vi "Print Main Screen.vi"(4 "Sample Rate in":T2=enum."500 Hz", 6 "Trigger Type in":T3(ring)=enum."Timed", 8 "Axis Names":string[](array[string]), 10 "Header Information in":T1, 11 "Graph Ref in":refnum<vi>) -> ()   [LabVIEW 2019]
uses:
  Type Defs and Controls/Header Information.ctl
  Type Defs and Controls/Sample Rates.ctl
panel:
  out "Time":string
  out "Date":string
  out "Legend":string[](array[string])
  out "Header Information":T1
  out "Sample Rate":T2=enum."500 Hz"
  out "Trigger Type":T3(ring)=enum."Timed"
  out "Graph":sgl[][](graph)
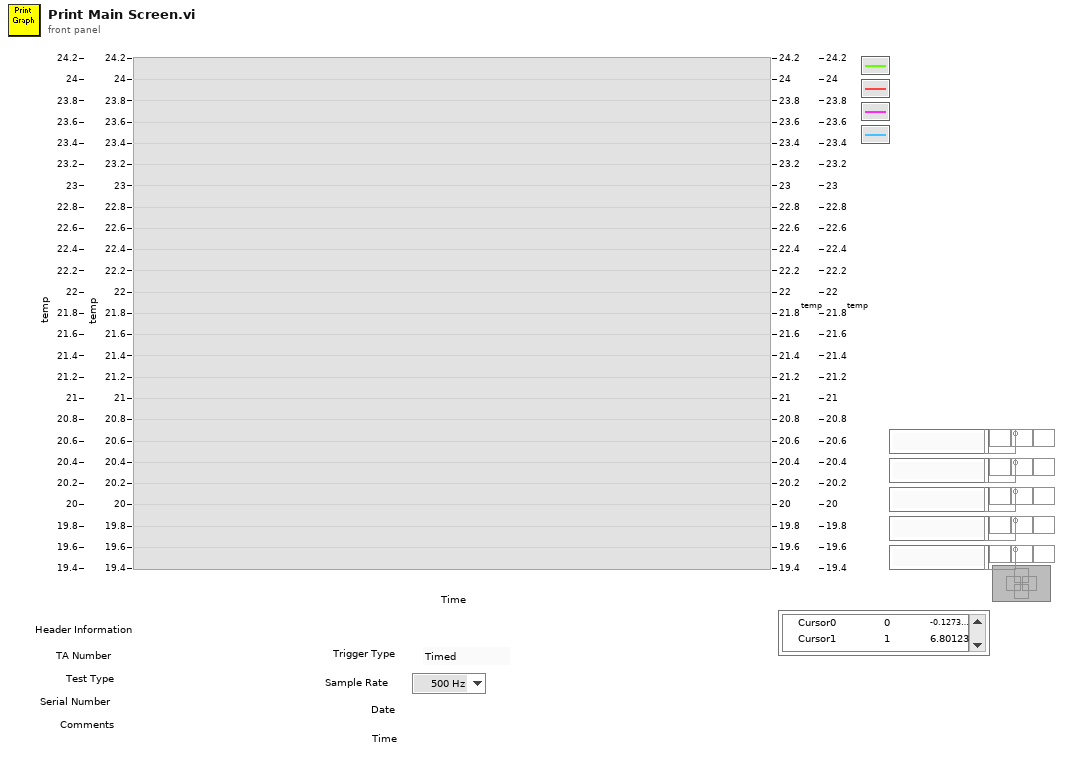
[diagram p1: front panel]
types:
  T1 = typedef "Header Information.ctl" = cluster{"TA Number":string, "Test Type":string, "Serial Number":string, "Comments":string}
  T2 = typedef "Sample Rates.ctl" = enum16{"2000 Hz", "1500 Hz", "1000 Hz", "500 Hz", "200 Hz", "100 Hz", "50 Hz", "25 Hz", "10 Hz", "1 Hz"}
  T3 = enum16{"Manual", "Timed", "Analog Rising", "Analog Falling"}
  T4 = typedef "LVFormatAndPrecisionTypeDef.ctl" = cluster{"Format":u8, "Precision":u8}
  T5 = typedef "LVRangeTypeDef.ctl" = cluster{"Minimum":dbl, "Maximum":dbl, "Increment":dbl, "Minor Increment":dbl, "Start":dbl}
  T6 = typedef "LVPointDoubleTypeDef.ctl" = cluster{"Cursor X":dbl, "Cursor Y":dbl}
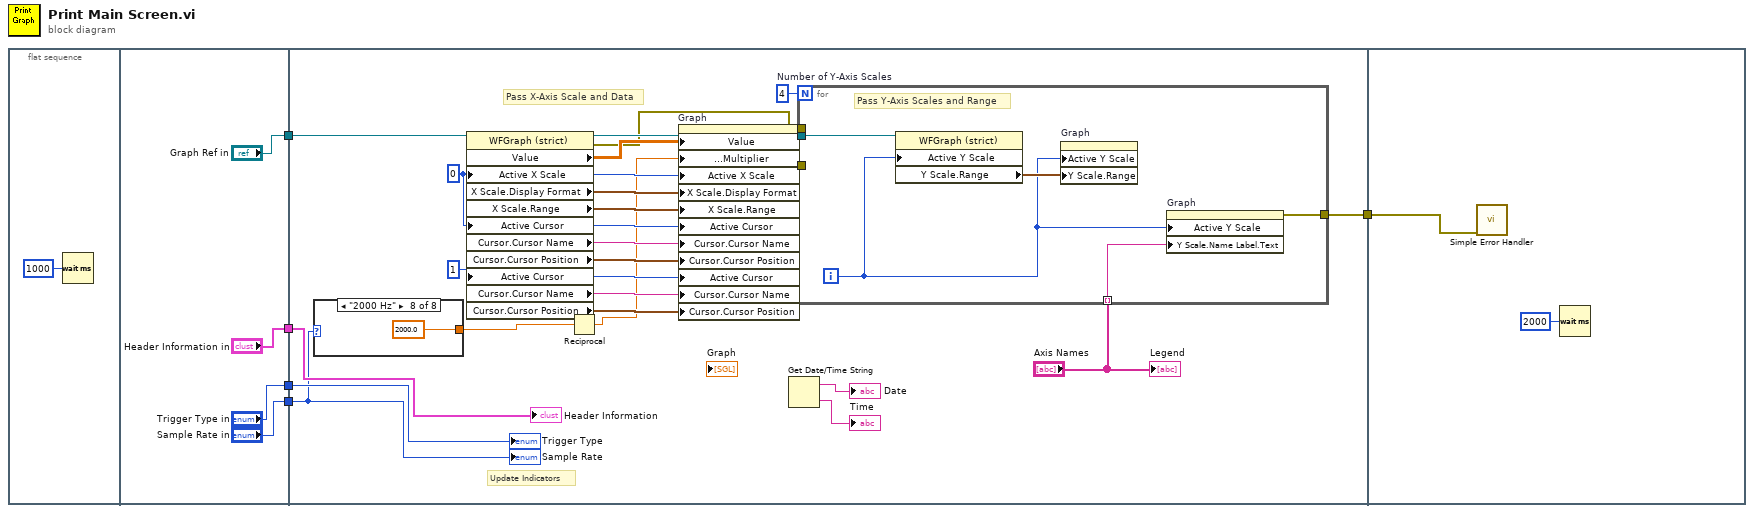
[diagram p0: block diagram]
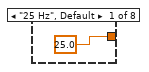
[diagram p2: hidden frame]
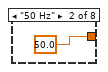
[diagram p3: hidden frame]
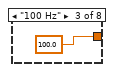
[diagram p4: hidden frame]
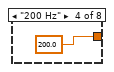
[diagram p5: hidden frame]
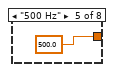
[diagram p6: hidden frame]
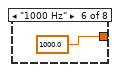
[diagram p7: hidden frame]
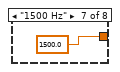
[diagram p8: hidden frame]
diagram:
  n1 = flat-sequence {
    tunnel: ["Graph Ref in"] -> w5
    tunnel: ["Header Information in"] -> w4
    tunnel: ["Trigger Type in"] -> w3
    tunnel: ["Sample Rate in"] -> w2
    tunnel: w5 -> [w33]
    tunnel: w4 -> [w21]
    tunnel: w3 -> [w29]
    tunnel: w2 -> [w20]
    tunnel: [w15] -> w1
    tunnel: w1 -> [w47]
    frame #0 {
      n2 = Wait (ms)(milliseconds to wait=u32 1000) -> ()  [unwired: 1 out]
    }
    frame #1 {
    }
    frame #2 {
      w24 = 1 ("Active X Scale")
      w28 = 4  # Number of Y-Axis Scales
      w27 = 0 ("Active X Scale")
      # "Update Indicators"
      # "Pass X-Axis Scale and Data"
      n3 = case shown="\"2000 Hz\"" w20 {
        tunnel: [sgl 25.0 ("scan rate (1000 scans/sec)") sgl 50.0 ("scan rate (1000 scans/sec)") sgl 100.0 ("scan rate (1000 scans/sec)") sgl 200.0 ("scan rate (1000 scans/sec)") sgl 500.0 ("scan rate (1000 scans/sec)") sgl 1000.0 ("scan rate (1000 scans/sec)") sgl 1500.0 ("scan rate (1000 scans/sec)") sgl 2000.0 ("scan rate (1000 scans/sec)")] -> w17
        frame "25 Hz", Default {
        }
        frame "50 Hz" {
        }
        frame "100 Hz" {
        }
        frame "200 Hz" {
        }
        frame "500 Hz" {
        }
        frame "1000 Hz" {
        }
        frame "1500 Hz" {
        }
        frame "2000 Hz" {
        }
      }
      n4 = property class="WFGraph (strict)"(reference=w33, "Active X Scale"=w27, "Active Cursor"=w27, "Active Cursor"=w24) -> (reference out=w32:refnum<vi>, error out=w12:errorcluster, "Value"=w13:sgl[][], "X Scale.Display Format"=w31:T4, "X Scale.Range"=w30:T5, "Cursor.Cursor Name"=w26:string, "Cursor.Cursor Position"=w25:T6, "Cursor.Cursor Name"=w23:string, "Cursor.Cursor Position"=w22:T6)  [unwired: 1 in]
      n5 = Reciprocal(x=w17) -> (1/x=w14:sgl)
      n6 = property on="Graph" class="WFGraph (strict)"("Value"=w13, "X Scale.Offset and Multiplier:Multiplier"=w14, "Active X Scale"=w27, "X Scale.Display Format"=w31, "X Scale.Range"=w30, "Active Cursor"=w27, "Cursor.Cursor Name"=w26, "Cursor.Cursor Position"=w25, "Active Cursor"=w24, "Cursor.Cursor Name"=w23, "Cursor.Cursor Position"=w22) -> (error out=w11:errorcluster)  [unwired: 2 in, 1 out]
      n7 = Get Date/Time String() -> (date string=→"Date":string, time string=→"Time":string)  [unwired: 3 in]
      n8 = for {
        N: w28 -> [_]
        tunnel: w32 -> [w44]
        tunnel: w12 -> [_]
        tunnel: "Axis Names" -> [w46] mode=indexing
        tunnel: [w45] -> w15
        tunnel: w11 -> [_]
        i -> [w42]
        # "Pass Y-Axis Scales and Range"
        n9 = property class="WFGraph (strict)"(reference=w44, "Active Y Scale"=w42) -> ("Y Scale.Range"=w43:T5)  [unwired: 1 in, 2 out]
        n10 = property on="Graph" class="WFGraph (strict)"("Active Y Scale"=w42, "Y Scale.Range"=w43) -> ()  [unwired: 2 in, 2 out]
        n11 = property on="Graph" class="WFGraph (strict)"("Active Y Scale"=w42, "Y Scale.Name Label.Text"=w46) -> (error out=w45:errorcluster)  [unwired: 2 in, 1 out]
      }
      "Header Information" <- w21
      "Trigger Type" <- w29
      "Sample Rate" <- w20
      "Legend" <- "Axis Names"
    }
    frame #3 {
      n12 = call <vilib>:"Simple Error Handler.vi"("error in (no error)"=w47) -> ()  [unwired: 4 in, 5 out]
      n13 = Wait (ms)(milliseconds to wait=u32 2000) -> ()  [unwired: 1 out]
    }
  }
